vi "Pattern recognition.vi"() -> ()   [LabVIEW 2015]
uses:
  <vilib>/vision/NI_Vision_Development_Module.lvlib
panel:
  in  "Template Path":path
  in  "Image Path":path
  out "Number of Matches Found":i32
  in  "Advanced Options":cluster{"Item":u16, "Value":dbl}[](array[cluster])=[{"Item"=1, "Value"=1.0}, {"Item"=103, "Value"=1.0}] {"Item" items=["LD Sampling - Minimum Constrast"=0, "LD Sampling - Enable Subpixel Accuracy"=1, "LD Sampling - Search Strategy"=2, "LD Sampling - Subpixel Iterations"=3, "LD Sampling - Subpixel Tolerance"=4, "LD Sampling - Initial Match List Length"=5, "LD Sampling - Match List Reduction Factor"=6, "LD Sampling - Initial Step Size"=7, "LD Sampling - Intermediate Angular Accuracy"=8, "-"=9, "Pyramid - Max Pyramid Level"=100, "Pyramid - Minimum Contrast"=102, "Pyramid - Enable Subpixel Accuracy"=103, "Pyramid - Subpixel Iterations"=104, "Pyramid - Subpixel Tolerance"=105, "Pyramid - Initial Match List Length"=106, "Pyramid - Match List Reduction Factor"=107, "Pyramid - Intermediate Angular Accuracy"=108, "Pyramid - Process Border Matches"=109, "Pyramid - Min Match Separation Distance"=111, "Pyramid - Min Match Separation Angle"=112, "Pyramid - Max Match Overlap"=113, "Pyramid - Max Cache in MB"=114, "Pyramid - Clear Cache"=115]}
  in  "Match Parameters":T1={"Number of Matches Requested"=1, "Minimum Match Score"=750.0, "Angle Ranges"=[]} {"Angle Ranges"."End Angle" min=-360 max=360; "Angle Ranges"."Start Angle" min=-360 max=360; "Minimum Match Score" min=0 max=1000; "Number of Matches Requested" min=1 max=9999}
  in  "Algorithm":i32(ring)=2 items=["All", "Low Discrepancy Sampling", "Grayscale Value Pyramid", "Gradients Pyramid"]
  out "Elapsed Time (ms)":dbl format="%.2f"
  out "Image":T2(plugin-control)
  out "Matches":T3(array[cluster]) {"Bounding Box"."y" format="%.2g"; "Bounding Box"."x" format="%.2g"; "Score" format="%.2f"; "Scale" format="%.2g"; "Angle" format="%.2g"; "Position"."y" format="%.2g"; "Position"."x" format="%.2g"}
  out "Template Report":T4={"Template Contrast"=0, "Grayvalue Max Pyramid Level"=-1, "Grayvalue Optimal Pyramid Level"=-1, "Gradient Max Pyramid Level"=-1, "Gradient Optimal Pyramid Level"=-1}
  out "Template":T2(plugin-control)
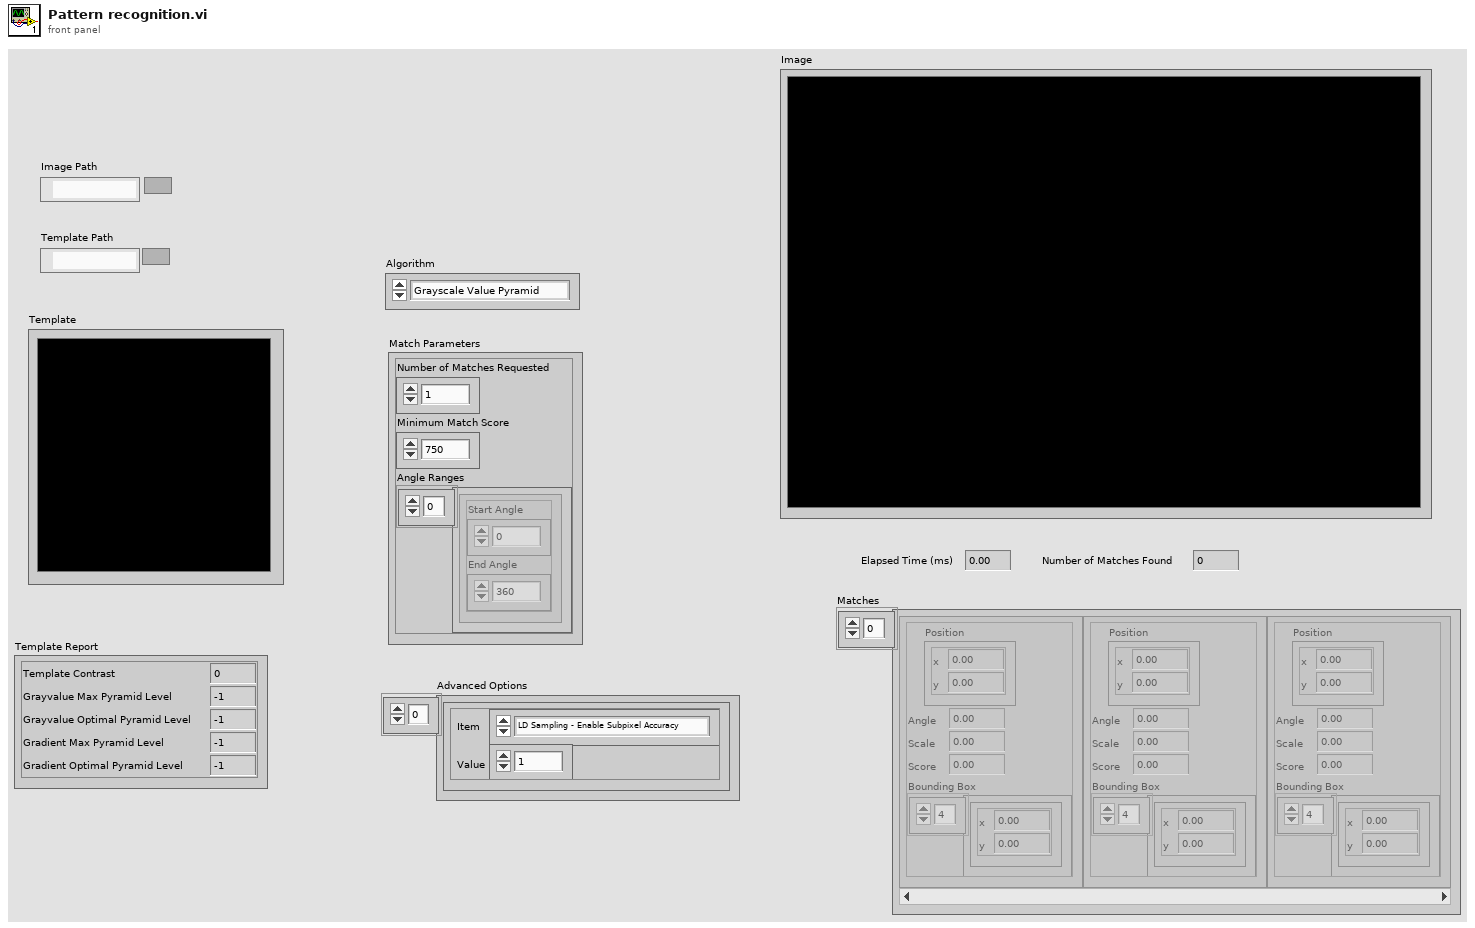
[diagram p1: front panel]
types:
  T1 = cluster{"Number of Matches Requested":i32, "Minimum Match Score":sgl, "Angle Ranges":cluster{"Start Angle":sgl, "End Angle":sgl}[]}
  T2 = typedef "IMAQ Image.ctl" = refnum<image>
  T3 = cluster{"Position":cluster{"x":sgl, "y":sgl}, "Angle":sgl, "Scale":sgl, "Score":sgl, "Bounding Box":cluster{"x":sgl, "y":sgl}[]}[]
  T4 = cluster{"Template Contrast":i32, "Grayvalue Max Pyramid Level":i32, "Grayvalue Optimal Pyramid Level":i32, "Gradient Max Pyramid Level":i32, "Gradient Optimal Pyramid Level":i32}
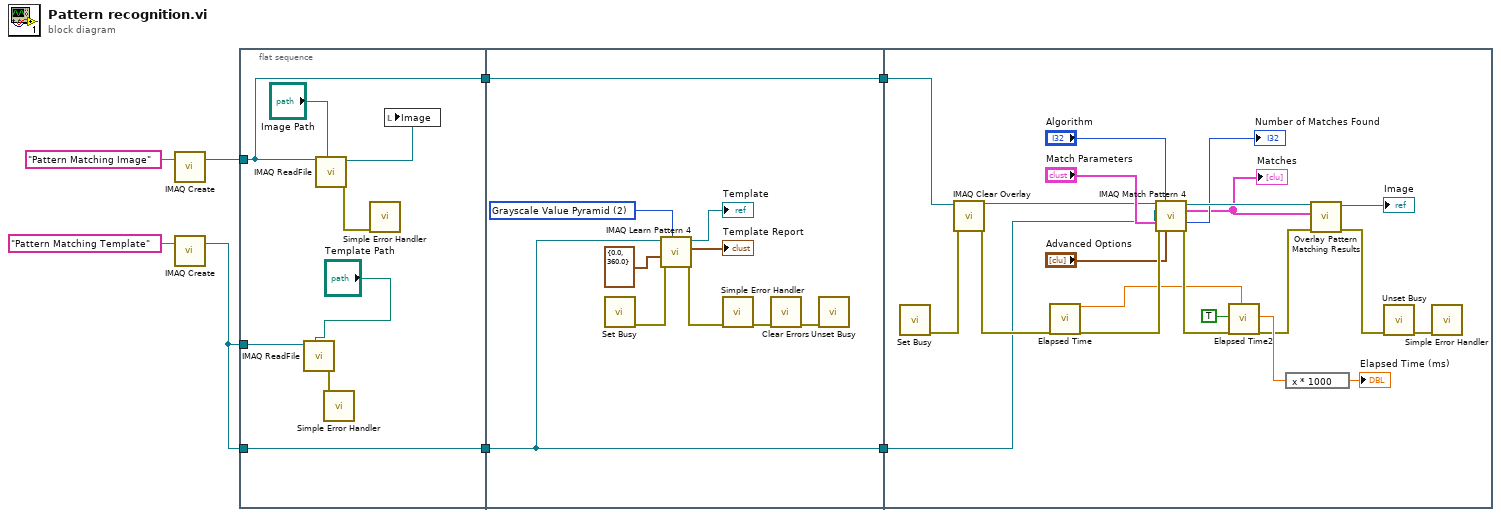
[diagram p0: block diagram]
diagram:
  n1 = call "IMAQ Create"("Image Name"="Pattern Matching Image") -> ("New Image"=w1:T2)  [unwired: 4 in, 1 out]
  n2 = call "IMAQ Create"("Image Name"="Pattern Matching Template") -> ("New Image"=w6:T2)  [unwired: 4 in, 1 out]
  n3 = flat-sequence {
    tunnel: w6 -> [w11]
    tunnel: w6 -> [w10]
    tunnel: [w10] -> w5
    tunnel: [w9] -> w3
    tunnel: w1 -> [w9]
    tunnel: w5 -> [w18]
    tunnel: [w18] -> w4
    tunnel: w3 -> [w17]
    tunnel: [w17] -> w2
    tunnel: w4 -> [w28]
    tunnel: w2 -> [w27]
    frame #0 {
      n4 = call "IMAQ ReadFile"("File Path"="Template Path", "Image"=w11) -> ("error out"=w15:errorcluster)  [unwired: 5 in, 4 out]
      n5 = call "IMAQ ReadFile"("File Path"="Image Path", "Image"=w9) -> ("error out"=w16:errorcluster, "Image Out"=w14:T2)  [unwired: 5 in, 3 out]
      n6 = call <vilib>:"Simple Error Handler.vi"("error in (no error)"=w15) -> ()  [unwired: 4 in, 5 out]
      n7 = call <vilib>:"Simple Error Handler.vi"("error in (no error)"=w16) -> ()  [unwired: 4 in, 5 out]
      n8 = local write "Image"(w14) -> ()
    }
    frame #1 {
      w26 = 2 items=["All", "Low Discrepancy Sampling", "Grayscale Value Pyramid", "Gradients Pyramid"] ("Algorithm")
      n9 = call <vilib>:"Set Busy.vi"() -> ("error out"=w23:errorcluster)  [unwired: 10 in, 1 out]
      n10 = call "IMAQ Learn Pattern 4"("Algorithm"=w26, "error in (no error)"=w23, "Angle Range"=cluster{"Start Angle":sgl, "End Angle":sgl} {"Start Angle"=0.0, "End Angle"=360.0}, "Image"=w18) -> ("error out"=w22:errorcluster, "Template Report"=→"Template Report":T4, "Template Image Out"=→"Template":T2)  [unwired: 5 in]
      n11 = call <vilib>:"Simple Error Handler.vi"("error in (no error)"=w22) -> ("error out"=w21:errorcluster)  [unwired: 4 in, 4 out]
      n12 = call <vilib>:"Clear Errors.vi"("error in (no error)"=w21) -> ("error out"=w20:errorcluster)  [unwired: 5 in, 1 out]
      n13 = call <vilib>:"Unset Busy.vi"("error in (no error)"=w20) -> ()  [unwired: 10 in, 1 out]
    }
    frame #2 {
      n14 = call <vilib>:"Set Busy.vi"() -> ("error out"=w41:errorcluster)  [unwired: 10 in, 1 out]
      n15 = call "IMAQ Clear Overlay"("error in (no error)"=w41, "Image"=w27) -> ("error out"=w38:errorcluster, "Image Out"=w42:T2)  [unwired: 8 in]
      n16 = call "Elapsed Time"("error in (no error)"=w38) -> ("Present (s)"=w33:dbl, "error out"=w37:errorcluster)  [unwired: 11 in, 6 out]
      n17 = call "IMAQ Match Pattern 4"("Image"=w42, "Algorithm"="Algorithm", "Template Image"=w28, "Parameters"="Match Parameters", "error in (no error)"=w37, "Advanced Options"="Advanced Options") -> ("Image (duplicate)"=w45:T2, "Matches (pixel)"=w29:T3, "Number of Matches"=→"Number of Matches Found":i32, "error out"=w36:errorcluster)  [unwired: 5 in, 1 out]
      "Matches" <- w29
      n18 = call "Elapsed Time2"("Reset"=TRUE, "error in (no error)"=w36, "Set Start Time (s)"=w33) -> ("Elapsed Time (s)"=w40:dbl, "error out"=w34:errorcluster)  [unwired: 9 in, 6 out]
      n19 = expression code="x * 1000"(w40) -> (→"Elapsed Time (ms)":dbl)
      n20 = call "Overlay Pattern Matching Results.vi"("error in"=w34, "Matches"=w29, "Image"=w45) -> ("error out"=w43:errorcluster, "Image Out"=→"Image":T2)  [unwired: 7 in]
      n21 = call <vilib>:"Unset Busy.vi"("error in (no error)"=w43) -> ("error out"=w32:errorcluster)  [unwired: 10 in]
      n22 = call <vilib>:"Simple Error Handler.vi"("error in (no error)"=w32) -> ()  [unwired: 4 in, 5 out]
    }
  }
